vi "Reset Position.vi"(8 "error in (no error)":errorcluster, 11 "Maxon Encoder in":refnum<class "Maxon Encoder.lvclass">) -> (0 "error out":errorcluster, 3 "Maxon Encoder out":refnum<class "Maxon Encoder.lvclass">)   [LabVIEW 2019, in "Maxon Encoder.lvclass"]
doc: "Resets the position of the encoder to 0."
uses:
  Maxon Encoder.lvclass
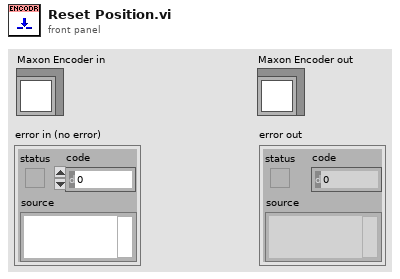
[diagram p1: front panel]
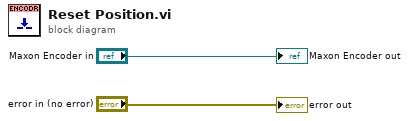
[diagram p0: block diagram]
diagram:
  "error out" <- "error in (no error)"
  "Maxon Encoder out" <- "Maxon Encoder in"
